vi "Read Diagram.vi"(9 "FlatSequenceFrame in":refnum<class "FlatSequenceFrame.lvclass">) -> (3 "FlatSequenceFrame out":refnum<class "FlatSequenceFrame.lvclass">, 4 "Diagram":refnum<class "Diagram.lvclass">)   [LabVIEW 2014, in "Raspberry Pi Compatible Compiler for LabVIEW.lvlib" / "FlatSequenceFrame.lvclass"]
uses:
  FlatSequenceFrame.lvclass
  Diagram/Diagram.lvclass
  FlatSequenceFrame.lvclass/FlatSequenceFrame.ctl
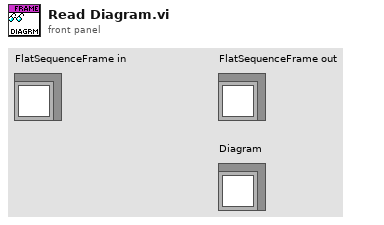
[diagram p1: front panel]
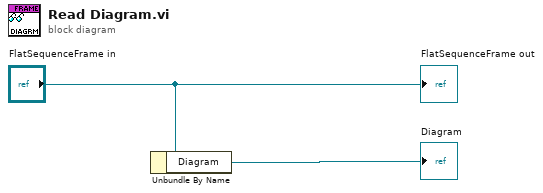
[diagram p0: block diagram]
diagram:
  n1 = Unbundle By Name("FlatSequenceFrame in") -> ("Diagram"=→"Diagram":refnum<class "Diagram.lvclass">)
  "FlatSequenceFrame out" <- "FlatSequenceFrame in"
